vi "RVC 2-link serial robot.vi"() -> ()   [LabVIEW 2013]
uses:
  <vilib>/Analysis/Matrix/Datatypes/RealMatrix.ctl
  <vilib>/robotics/Kinematics/Analytical/Initialize Generic Serial Arm.vi
  <vilib>/robotics/Kinematics/Analytical/NI_Robotics_AnalyticKinematics.lvlib
  <vilib>/robotics/Kinematics/Robot/NI_Robotics_Serial Robot Arm.lvclass
  <vilib>/Analysis/Matrix/NI_Matrix.lvlib
panel:
  out "transformation":picture
  out "forward kinematics":T1
  out "3D Picture":refnum<vi>(3d-picture)
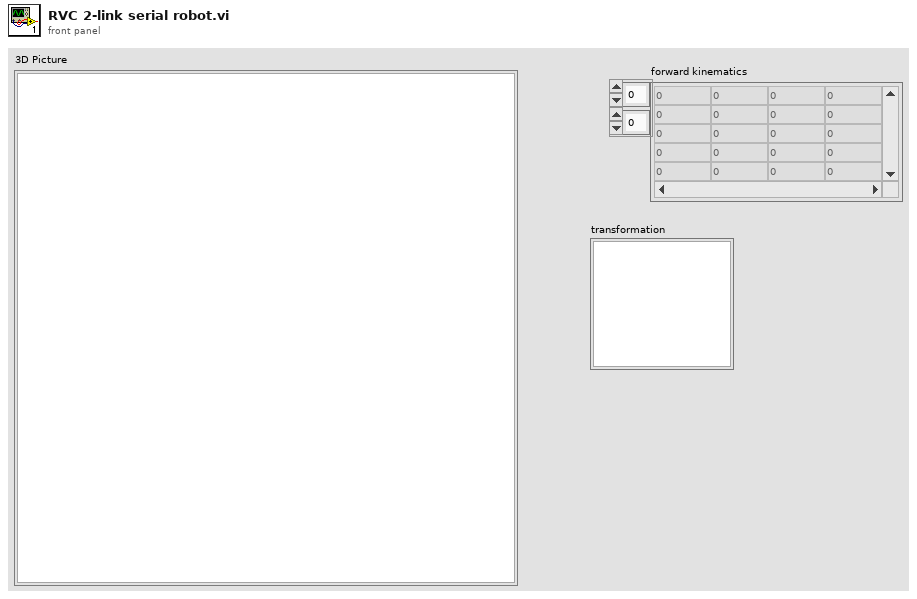
[diagram p1: front panel]
types:
  T1 = typedef "NI_Matrix.lvlib/RealMatrix.ctl" = dbl[][]
  T2 = typedef "DH Kinematic Parameters.ctl" = cluster{"twist angle":dbl, "length":dbl, "rotation angle":dbl, "offset distance":dbl, "joint type":T3, "joint coordinate offset":dbl}
  T3 = typedef "NI_Robotics_Link.lvclass/Joint Type.ctl" = enum16{"Revolute", "Prismatic"}
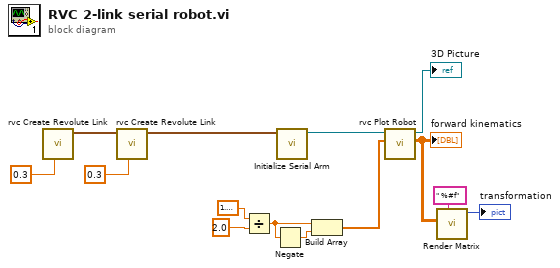
[diagram p0: block diagram]
diagram:
  n1 = call "rvc Create Revolute Link.vi"("length (a)"=0.3) -> ("Array"=w6:T2[])  [unwired: 10 in]
  n2 = call "rvc Create Revolute Link.vi"("length (a)"=0.3, "Array 2"=w6) -> ("Array"=w14:T2[])  [unwired: 9 in]
  n3 = Divide(x=1.5707963267948966, y=2.0) -> (x/y=w9:dbl)
  n4 = Negate(x=w9) -> (-x=w8:dbl)
  n5 = call-poly <vilib>:"Initialize Serial Arm.vi"("kinematic parameters"=w14) -> ("serial arm out"=w13:refnum<class "NI_Robotics_Serial Robot Arm.lvclass">)  [unwired: 9 in, 1 out]
  n6 = Build Array(w9, w8) -> (w7:dbl[])
  n7 = call "rvc Plot Robot.vi"("joint positions"=w7, "NI_Robotics_Serial Robot Arm in"=w13) -> ("forward kinematics"=w1:T1, "Scene Object Out"=→"3D Picture":refnum<vi>)  [unwired: 8 in]
  "forward kinematics" <- w1
  n8 = call "Render Matrix.vi"("format string"=" %#f", "A"=w1) -> ("picture out"=→"transformation":picture)  [unwired: 9 in]
